vi "Check Bounds (Power of 2).vi"(5 "source vi name":string, 6 "count power of 2":i16, 7 "buffer count":u64 format="%d elements", 8 "error in (no error)":errorcluster, 9 "offset (0)":u64 format="%d bytes", 10 "move count":u64 format="%d elements", 11 "Pointer in":refnum<class "Pointer.lvclass">) -> (0 "error out":errorcluster, 1 "offset":u64 format="%d bytes", 2 "move count":u64 format="%d elements", 3 "Pointer out":refnum<class "Pointer.lvclass">)   [LabVIEW 2020, in "Memory Manager.lvlib" / "Pointer.lvclass"]
uses:
  Pointer.lvclass
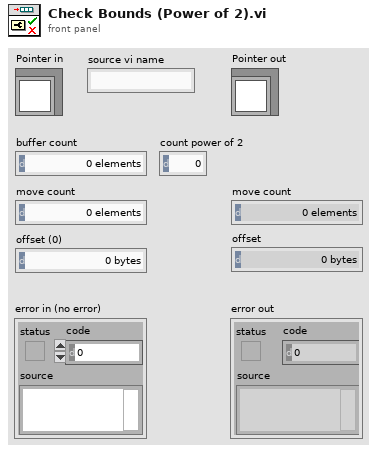
[diagram p1: front panel]
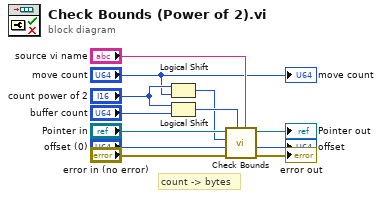
[diagram p0: block diagram]
diagram:
  # "count -> bytes"
  n1 = Logical Shift(y="count power of 2", x="move count") -> (x << y=w1:u64)
  n2 = Logical Shift(y="count power of 2", x="buffer count") -> (x << y=w10:u64)
  n3 = call "Check Bounds.vi"("source vi name"="source vi name", "buffer size"=w10, "error in (no error)"="error in (no error)", "offset (0)"="offset (0)", "size to move"=w1, "Pointer in"="Pointer in") -> ("error out"=→"error out":errorcluster, "offset"=→"offset":u64, "Pointer out"=→"Pointer out":refnum<class "Pointer.lvclass">)  [unwired: 2 in, 1 out]
  "move count" <- "move count"
